vi "Measurement UI.vi"() -> ()   [LabVIEW 2024, in "Averaged - Broadband UI.lvlib"]
uses:
  Averaged - Broadband UI.lvlib
panel:
  out "COH":cluster{"f0":dbl, "df":dbl, "coherence":dbl[]}(graph)
  in  "ai response terminal configuration":i32=-1
  in  "ai response range":dbl=3.16 format="± %#_6f V"
  in  "ai response channel":string="Dev1/ai1"
  in  "ai reference terminal configuration":i32=-1
  in  "ai ref range":dbl=3.16 format="± %#_6f V"
  in  "ai reference channel":string="Dev1/ai0"
  in  "ao terminal configuration":i32=-1
  in  "ao range":dbl=3.16 format="± %#_4f V"
  in  "ao stimulus channel":string="Dev1/ao0"
  out "phase":dbl[](array[numeric])
  out "magnitude":dbl[](array[numeric])
  out "coherence":dbl[](array[numeric])
  out "df":dbl format="%#_13g"
  out "f0":dbl format="%#_13g"
  out "MAG":cluster{"f0":dbl, "df":dbl, "magnitude":dbl[]}(graph)
  out "PHI":cluster{"f0":dbl, "df":dbl, "phase":dbl[]}(graph)
  out "FRF file path":path caption="frequency response file path"
  in  "ai response":T1={"ai response channel (I/O)"="", "range"=3.16, "terminal configuration"=-1} {"terminal configuration" items=["Default"=-1, "RSE"=10083, "NRSE"=10078, "Differential"=10106, "Pseudodifferential"=12529]; "range" format="± %#_6f V"}
  in  "ai reference":T2={"ai reference channel (I/O)"="", "range"=3.16, "terminal configuration"=-1} {"terminal configuration" items=["Default"=-1, "RSE"=10083, "NRSE"=10078, "Differential"=10106, "Pseudodifferential"=12529]; "range" format="± %#_6f V"}
  in  "ao stimulus":T3={"ao stimulus channel (I/O)"="", "range"=3.16, "terminal configuration"=-1} {"terminal configuration" items=["Default"=-1, "RSE"=10083, "Differential"=10106, "Pseudodifferential"=12529]; "range" format="± %#_4f V"}
  in  "sample rate":dbl=51200.0 format="%#_4p Hz"
  in  "signal type":i32(ring)=1 items=["Uniform white noise", "Gaussian white noise", "Pink noise", "Periodic random noise"]
  in  "level":dbl=0.4 format="%#_6f V"
  in  "averaging mode":i32(ring)=2 items=["No averaging", "Vector averaging", "RMS averaging", "Peak hold"]
  in  "frequency resolution":dbl=10.0 format="%#_4f Hz"
  in  "averages":i32=20 min=1
  out "averages completed":dbl
  # "DAQ"
  # "Source"
  # "Measurement"
  # "Status"
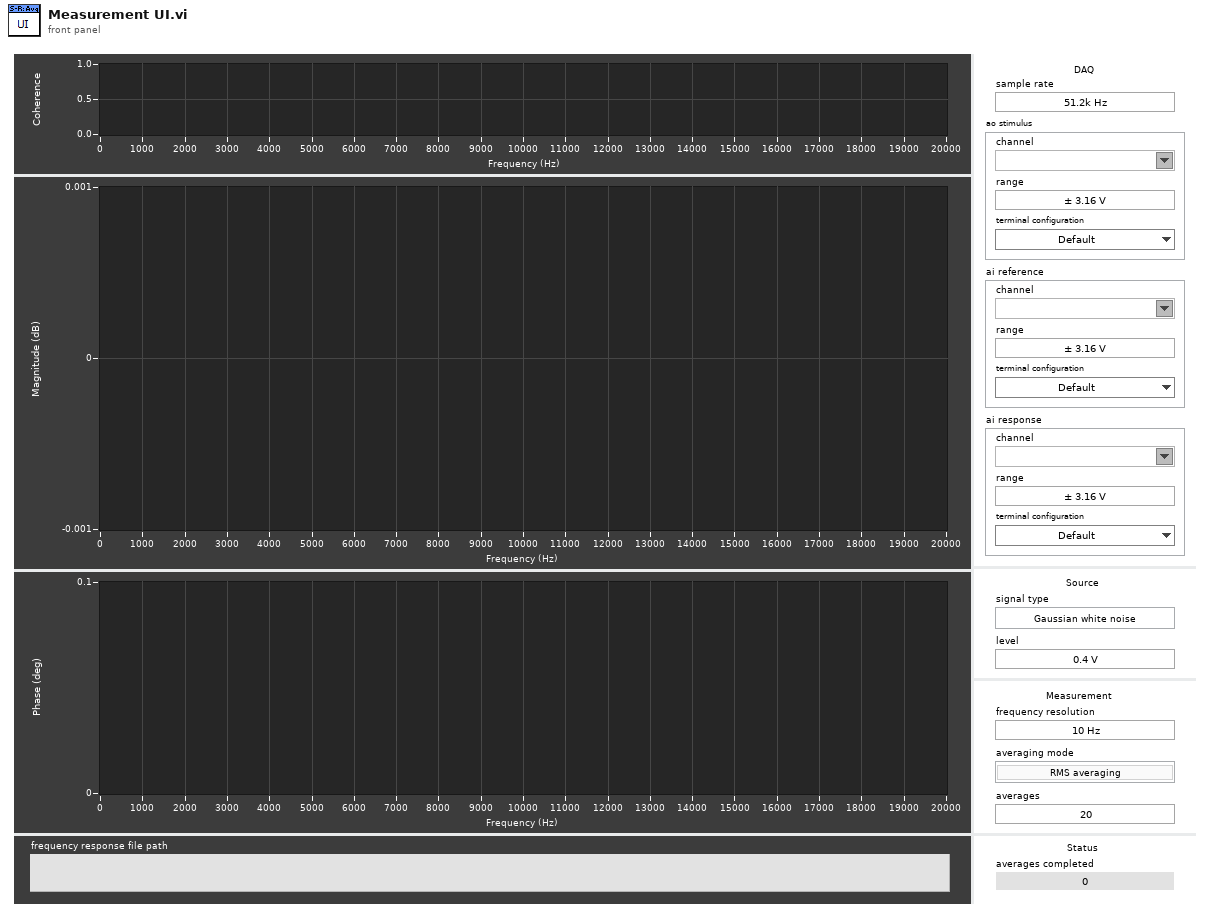
[diagram p1: front panel]
types:
  T1 = cluster{"ai response channel (I/O)":tag, "range":dbl, "terminal configuration":i32}
  T2 = cluster{"ai reference channel (I/O)":tag, "range":dbl, "terminal configuration":i32}
  T3 = cluster{"ao stimulus channel (I/O)":tag, "range":dbl, "terminal configuration":i32}
  T4 = enum8{"Enabled", "Disabled", "Disabled and Grayed Out"}
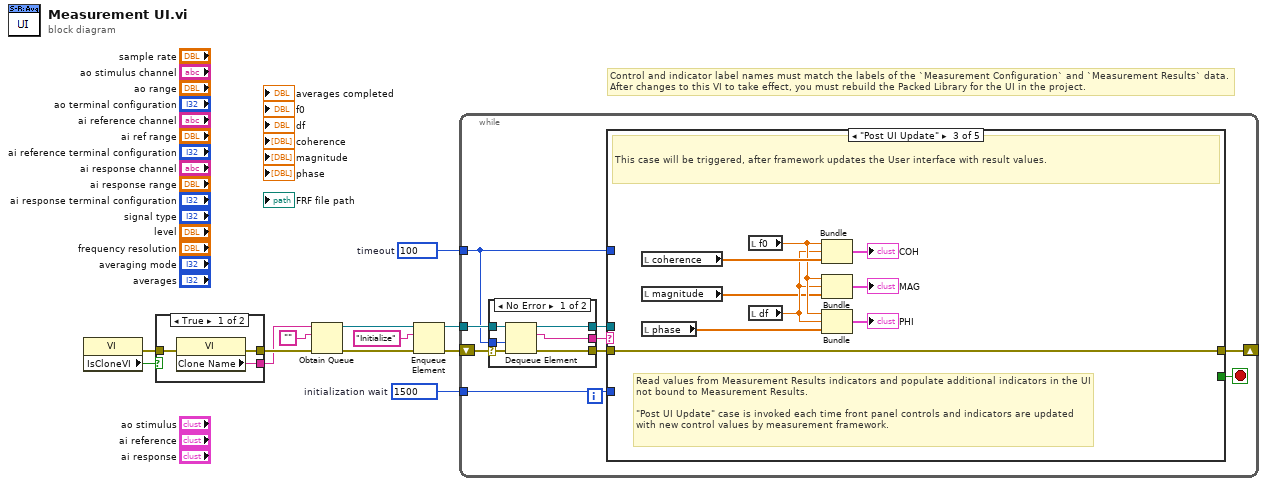
[diagram p0: block diagram]
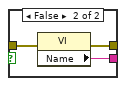
[diagram p2: hidden frame]
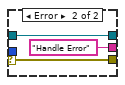
[diagram p3: hidden frame]
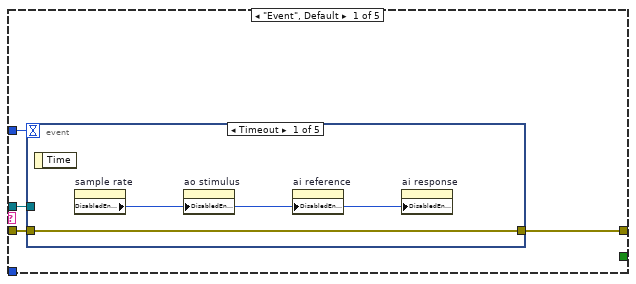
[diagram p4: hidden frame]
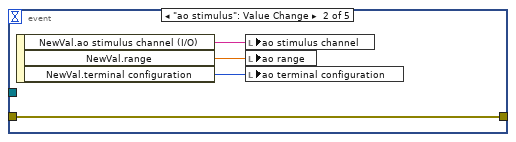
[diagram p5: hidden frame]
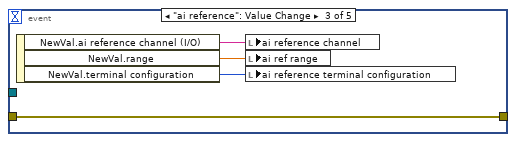
[diagram p6: hidden frame]
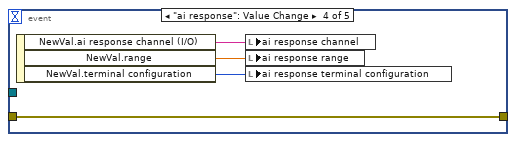
[diagram p7: hidden frame]
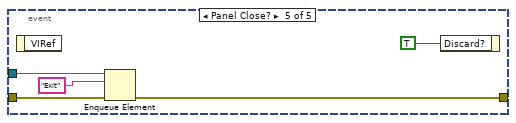
[diagram p8: hidden frame]
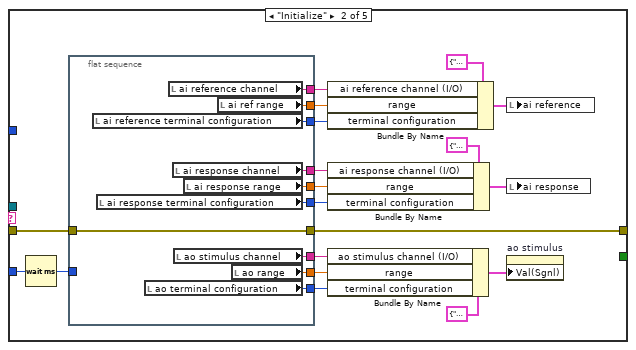
[diagram p9: hidden frame]
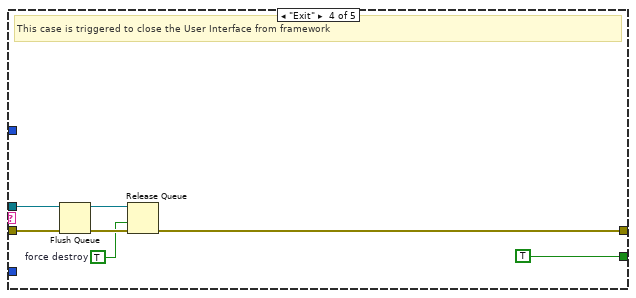
[diagram p10: hidden frame]
diagram:
  w1 = u32 1500  # initialization wait
  w2 = 100  # timeout
  # "Control and indicator label names must match the labels of the `Measurement Configuration` and `Measurement Results` data. \nAfter changes to this VI to take effect, you must rebuild the Packed Library for the UI in the project."
  n1 = property class="VI"() -> (error out=w3:errorcluster, "IsCloneVI"=w4:bool)  [unwired: 2 in, 1 out]
  n2 = case shown="True" w4 {
    tunnel: [w15 w18] -> w12
    tunnel: [w14 w17] -> w11
    tunnel: w3 -> [w13 w16]
    frame True {
      n3 = property class="VI"(error in=w13) -> (error out=w15:errorcluster, "Clone Name"=w14:string)  [unwired: 1 in, 1 out]
    }
    frame False {
      n4 = property class="VI"(error in=w16) -> (error out=w18:errorcluster, "Name"=w17:string)  [unwired: 1 in, 1 out]
    }
  }
  n5 = Obtain Queue(name (unnamed)=w11, element data type="", error in (no error)=w12) -> (queue out=w8:refnum<queue>, error out=w10:errorcluster)  [unwired: 2 in, 1 out]
  n6 = Enqueue Element(queue=w8, element="Initialize", error in (no error)=w10) -> (queue out=w7:refnum<queue>, error out=w9:errorcluster)  [unwired: 1 in, 1 out]
  n7 = while {
    shift-right: [w22] -> _
    shift-left: w9 -> [w27]
    tunnel: w7 -> [w25]
    tunnel: w2 -> [w20]
    tunnel: w1 -> [w19]
    stop <- w21 stop-if-true
    n8 = case shown="No Error" w27 {
      selector: w27 -> [w33 w36]
      tunnel: [w32 w36] -> w26
      tunnel: w25 -> [w31 w35]
      tunnel: [w30 w35] -> w24
      tunnel: [w29 "Handle Error"] -> w23
      tunnel: w20 -> [w28 _]
      frame No Error {
        n9 = Dequeue Element(queue=w31, timeout in ms (-1)=w28, error in (no error)=w33) -> (queue out=w30:refnum<queue>, element=w29:string, error out=w32:errorcluster)  [unwired: 1 out]
      }
      frame Error {
      }
    }
    n10 = case shown="\"Post UI Update\"" w23 {
      tunnel: w26 -> [w39 w76 w97 w104 w105]
      tunnel: w24 -> [w38 _ _ w102 _]
      tunnel: [w40 w77 w97 w99 w105] -> w22
      tunnel: [_ _ _ TRUE _] -> w21
      tunnel: w20 -> [w37 _ _ _ _]
      tunnel: w19 -> [_ w78 _ _ _]
      frame "Event", Default {
        n11 = event shown="[0] Timeout" {
          selector: _ -> [_ _ _ _ _]
          dyn-events: _ -> [_ _ _ _ _]
          timeout: w37 -> [_ _ _ _ _]
          tunnel: [w42 w43 w47 w54 w57] -> w40
          tunnel: w39 -> [w42 w43 w47 w54 w58]
          tunnel: w38 -> [_ _ _ _ w56]
          event Timeout {
            n12 = event-data() -> ()  [unwired: 1 in, 1 out]
            n13 = property on="sample rate" class="DigNum (strict)"() -> ("DisabledEnum"=w41:T4)  [unwired: 2 in, 2 out]
            n14 = property on="ao stimulus" class="Clust (strict)"("DisabledEnum"=w41) -> ()  [unwired: 2 in, 2 out]
            n15 = property on="ai reference" class="Clust (strict)"("DisabledEnum"=w41) -> ()  [unwired: 2 in, 2 out]
            n16 = property on="ai response" class="Clust (strict)"("DisabledEnum"=w41) -> ()  [unwired: 2 in, 2 out]
          }
          event "ao stimulus": Value Change {
            n17 = event-data() -> ("NewVal.ao stimulus channel (I/O)"=w46:tag, "NewVal.range"=w45:dbl, "NewVal.terminal configuration"=w44:i32)  [unwired: 1 in]
            n18 = local write "ao stimulus channel"(w46) -> ()
            n19 = local write "ao range"(w45) -> ()
            n20 = local write "ao terminal configuration"(w44) -> ()
          }
          event "ai reference": Value Change {
            n21 = event-data() -> ("NewVal.ai reference channel (I/O)"=w50:tag, "NewVal.range"=w49:dbl, "NewVal.terminal configuration"=w48:i32)  [unwired: 1 in]
            n22 = local write "ai reference channel"(w50) -> ()
            n23 = local write "ai ref range"(w49) -> ()
            n24 = local write "ai reference terminal configuration"(w48) -> ()
          }
          event "ai response": Value Change {
            n25 = event-data() -> ("NewVal.ai response channel (I/O)"=w53:tag, "NewVal.range"=w52:dbl, "NewVal.terminal configuration"=w51:i32)  [unwired: 1 in]
            n26 = local write "ai response channel"(w53) -> ()
            n27 = local write "ai response range"(w52) -> ()
            n28 = local write "ai response terminal configuration"(w51) -> ()
          }
          event Panel Close? {
            n29 = event-data() -> ()  [unwired: 1 in, 1 out]
            n30 = Enqueue Element(queue=w56, element="Exit", error in (no error)=w58) -> (error out=w57:errorcluster)  [unwired: 1 in, 2 out]
            n31 = event-data("Discard?"=TRUE) -> ()  [unwired: 1 in, 1 out]
          }
        }
      }
      frame "Initialize" {
        n32 = Wait (ms)(milliseconds to wait=w78) -> (millisecond timer value=w70:u32)
        n33 = flat-sequence {
          tunnel: [w88] -> w77
          tunnel: w76 -> [w88]
          tunnel: [w87] -> w74
          tunnel: [w86] -> w73
          tunnel: [w85] -> w72
          tunnel: w70 -> [_]
          tunnel: [w84] -> w68
          tunnel: [w83] -> w67
          tunnel: [w82] -> w66
          tunnel: [w81] -> w65
          tunnel: [w80] -> w63
          tunnel: [w79] -> w62
          frame #0 {
            n34 = local read "ai reference terminal configuration"() -> (w82:i32)
            n35 = local read "ai response terminal configuration"() -> (w81:i32)
            n36 = local read "ao terminal configuration"() -> (w85:i32)
            n37 = local read "ai reference channel"() -> (w84:string)
            n38 = local read "ai response channel"() -> (w79:string)
            n39 = local read "ao stimulus channel"() -> (w87:string)
            n40 = local read "ai response range"() -> (w80:dbl)
            n41 = local read "ai ref range"() -> (w83:dbl)
            n42 = local read "ao range"() -> (w86:dbl)
          }
        }
        n43 = Bundle By Name(cluster=T2 {"ai reference channel (I/O)"="", "range"=3.16, "terminal configuration"=-1} ("ai reference"), "ai reference channel (I/O)"=w68, "range"=w67, "terminal configuration"=w66) -> (w61:T2)
        n44 = Bundle By Name(cluster=T1 {"ai response channel (I/O)"="", "range"=3.16, "terminal configuration"=-1} ("ai response"), "ai response channel (I/O)"=w62, "range"=w63, "terminal configuration"=w65) -> (w60:T1)
        n45 = Bundle By Name(cluster=T3 {"ao stimulus channel (I/O)"="", "range"=3.16, "terminal configuration"=-1} ("ao stimulus"), "ao stimulus channel (I/O)"=w74, "range"=w73, "terminal configuration"=w72) -> (w71:T3)
        n46 = local write "ai reference"(w61) -> ()
        n47 = local write "ai response"(w60) -> ()
        n48 = property on="ao stimulus" class="Clust (strict)"("Val(Sgnl)"=w71) -> ()  [unwired: 2 in, 2 out]
      }
      frame "Post UI Update" {
        # "Read values from Measurement Results indicators and populate additional indicators in the UI not bound to Measurement Results.\n\n\"Post UI Update\" case is invoked each time front panel controls and indicators are updated with new control values by measurement framework."
        # "This case will be triggered, after framework updates the User interface with result values."
        n49 = local read "coherence"() -> (w96:dbl[])
        n50 = local read "magnitude"() -> (w93:dbl[])
        n51 = local read "phase"() -> (w92:dbl[])
        n52 = local read "f0"() -> (w95:dbl)
        n53 = local read "df"() -> (w94:dbl)
        n54 = Bundle("f0"=w95, "df"=w94, "coherence"=w96) -> (→"COH":cluster{"f0":dbl, "df":dbl, "coherence":dbl[]})  [unwired: 1 in]
        n55 = Bundle("f0"=w95, "df"=w94, "magnitude"=w93) -> (→"MAG":cluster{"f0":dbl, "df":dbl, "magnitude":dbl[]})  [unwired: 1 in]
        n56 = Bundle("f0"=w95, "df"=w94, "phase"=w92) -> (→"PHI":cluster{"f0":dbl, "df":dbl, "phase":dbl[]})  [unwired: 1 in]
      }
      frame "Exit" {
        w98 = TRUE  # force destroy
        # "This case is triggered to close the User Interface from framework"
        n57 = Flush Queue(queue=w102, error in (no error)=w104) -> (queue out=w101:refnum<queue>, error out=w100:errorcluster)  [unwired: 1 out]
        n58 = Release Queue(queue=w101, force destroy? (F)=w98, error in (no error)=w100) -> (error out=w99:errorcluster)  [unwired: 2 out]
      }
      frame "Handle Error" {
      }
    }
  }
